vi "SwitchesMirrors Loop.vi"(6 "Used functions":bool, 8 "error in":errorcluster, 9 "IBM OptoElectroMechanics Configuration":T1={"Parameter Analizer"={"Parameter Analyzer VISA Session"="COM1", "Sweeping Time Parameters"={"Integration Time"=0, "Short Integration Time (s)"=1.0, "Long Integration Time (s)"=0.0, "Wait Time Parameter"=1.0}, "Acquisition Mode"=enum."Sweeping Mode", "Status Polling Time (ms)"=0, "Comment"="Test VI", "SMU 1 - Sweeping"={"Start / Offset"=0.0, "Stop / Ratio"=1.0, "Step \n(linear only)"=0.01, "Compliance"=0.1, "Power \nCompliance"=0.0, "Mode"=0, "Function"=0, "Sweep Mode"=FALSE}, "SMU 2 - Sweeping"={"Start / Offset"=0.0, "Stop / Ratio"=1.0, "Step \n(linear only)"=0.01, "Compliance"=0.1, "Power \nCompliance"=0.0, "Mode"=0, "Function"=0, "Sweep Mode"=FALSE}, "SMU 3 - Sweeping"={"Start / Offset"=0.0, "Stop / Ratio"=1.0, "Step \n(linear only)"=0.01, "Compliance"=0.1, "Power \nCompliance"=0.0, "Mode"=0, "Function"=0, "Sweep Mode"=FALSE}, "SMU 4 - Sweeping"={"Start / Offset"=0.0, "Stop / Ratio"=1.0, "Step \n(linear only)"=0.01, "Compliance"=0.1, "Power \nCompliance"=0.0, "Mode"=0, "Function"=0, "Sweep Mode"=FALSE}, "Sweep Spacing"=0, "Range"=0, "SMU1 - Sampling"={"Source"=10.0, "Compliance"=1e-05, "Mode"=0, "Function"=FALSE}, "SMU2 - Sampling"={"Source"=1.0, "Compliance"=1.0, "Mode"=0, "Function"=FALSE}, "SMU3 - Sampling"={"Source"=10.0, "Compliance"=1e-05, "Mode"=0, "Function"=FALSE}, "SMU4 - Sampling"={"Source"=0.1, "Compliance"=60.0, "Mode"=10, "Function"=FALSE}, "Sampling Time Parameters"={"Initial Interval (s)"=0.1, "Number of Samples"=60, "Total Sampling Time (s)"=10.0, "Hold Time (s)"=0.0, "Sampling Mode"=0, "Sampling Time"=0}, "Stop Condition"={"Enable Delay (s)"=0.0, "Name"="", "Threshold"=0.0, "num. of events"=1, "Event"=0, "Stop Condition Enable"=FALSE}}, "Switching Matrix"={"Switching Matrix VISA Session"="GPIB0::18::INSTR", "Connections"=[{"Connections"=[FALSE, FALSE, FALSE, FALSE, FALSE, FALSE, FALSE, FALSE, FALSE, FALSE, FALSE, FALSE], "Connection Type"=enum."Disconnected"}, {"Connections"=[FALSE, FALSE, FALSE, FALSE, FALSE, FALSE, FALSE, FALSE, FALSE, FALSE, FALSE, FALSE], "Connection Type"=enum."Disconnected"}, {"Connections"=[FALSE, FALSE, FALSE, FALSE, FALSE, FALSE, FALSE, FALSE, FALSE, FALSE, FALSE, FALSE], "Connection Type"=enum."Disconnected"}, {"Connections"=[FALSE, FALSE, FALSE, FALSE, FALSE, FALSE, FALSE, FALSE, FALSE, FALSE, FALSE, FALSE], "Connection Type"=enum."Disconnected"}, {"Connections"=[FALSE, FALSE, FALSE, FALSE, FALSE, FALSE, FALSE, FALSE, FALSE, FALSE, FALSE, FALSE], "Connection Type"=enum."Disconnected"}, {"Connections"=[FALSE, FALSE, FALSE, FALSE, FALSE, FALSE, FALSE, FALSE, FALSE, FALSE, FALSE, FALSE], "Connection Type"=enum."Disconnected"}, {"Connections"=[FALSE, FALSE, FALSE, FALSE, FALSE, FALSE, FALSE, FALSE, FALSE, FALSE, FALSE, FALSE], "Connection Type"=enum."Disconnected"}, {"Connections"=[FALSE, FALSE, FALSE, FALSE, FALSE, FALSE, FALSE, FALSE, FALSE, FALSE, FALSE, FALSE], "Connection Type"=enum."Disconnected"}]}, "Stress Control"={"Stress Control VISA Session"="StrainMotor", "Axis"=0, "Motion"=0, "Destination (°)"=0.0, "Speed (°/s)"=4.0, "Position (°)"=25.0}, "Optical Spectrometer"={"Laser Settings"={"Laser Wavelength"=enum."365 nm", "Neutral Density Filter"=enum."100%"}, "Spectrometer Settings"={"Confocal Hole Size (µm)"=0.0, "Grating"=2, "Detector"=enum."InGaAs Array"}, "Acquisition Settings"={"Acquisition Mode"=enum."Multi-Window", "Spectal Position (nm)"=632.0, "From (nm)"=735.0, "To (nm)"=0.0, "Integration Time (s)"=0.0, "Number of Accumulations"=3, "AutoScanning"=FALSE, "Spike Removal"=FALSE}, "Path"=path "C:/07 - Prizes and Awards/Marie Curie Prize/Reply Editors Final NCOMMS(10).docx"}, "Switches & Mirrors"={"Relay VISA Session"="COM1", "Switches"={"Laser"=FALSE, "Video"=FALSE}, "Delays (ms)"={"Laser"=500, "Video"=1500}}, "Camera"={"Settings"={"Pixel clock"=20, "Frame rate"=30.0, "Exposure time"=33.21525, "Master Gain"=0, "Red Gain"=0, "Green Gain"=0, "Blue Gain"=0, "Auto Gain"=FALSE, "White-balance"=FALSE, "Color Correction"=FALSE}}, "XYZ Stage"={"Connection Settings"={"Tango VISA"="", "Baudrate"=57600, "Show Protocol?"=FALSE}, "Manual Control"={"North"=FALSE, "South"=FALSE, "West"=FALSE, "East"=FALSE, "Up"=FALSE, "Down"=FALSE, "Stop"=FALSE, "XY Step"=0.0, "Z step"=0.0}, "Coordinate Control"={"Motion Mode"=enum."Absolute", "Destination [mm]"=[]}}, "AutoFocus"={"Matching Criteria"={"Minimum Score"=700.0, "Color Score Weight"=700.0, "Minimum Contrast"=50, "Match Mode"=0, "Match Feature Mode"=0, "Subpixel Accuracy"=TRUE, "Color Sensitivity"=1, "Search Strategy"=1}, "Z Scan Parameters"={"Z Range"=1380.0, "Resolution"=5000.0, "Initial Direction"=enum."Up", "Focus Threshold"=0.1, "Ascent Constant"=0.1}, "Displacement"=0.0, "Transformation Matrix"=[]}, "Sava Data"={"Workspace Info"={"Device Name"="ProberHead_Tst_C29K3_7(2)", "Device Info"="ProberHead_Tst_C29", "Path"=path "C:/Users/gio/Desktop/ProbeHeadTest"}, "Instrument Configuration"={"Instrument"=enum."Unknown Instrument", "Configuration"="Test Configuration"}, "Stress Motor Position"=0.0, "Electrical Measurement"={"Sequence"=[], "V1"=[], "V2"=[], "V3"=[], "V4"=[], "I1"=[], "I2"=[], "I3"=[], "I4"=[]}, "Optical Spectrum"={"Intensity"=[], "Wavelength"=[], "Energy"=[], "Raman Shift"=[], "Detector Temperature"=0.0}}, "PlotData"={"Sliders"={"Strain Sequence"=0, "Instrument Sequence"=0}, "Measurement"={"Which Instrument?"=enum."No Plot", "Electrical Measurement"={"Sequence"=[], "V1"=[], "V2"=[], "V3"=[], "V4"=[], "I1"=[], "I2"=[], "I3"=[], "I4"=[]}, "Measurement Mode"=enum."Sweeping Mode", "Optical Spectrum"={"Intensity"=[], "Wavelength"=[], "Energy"=[], "Raman Shift"=[], "Detector Temperature"=0.0}}, "Instrument Steps"=[], "Strain Points"=[]}, "Instrument Sequence"={"Caller VI"=enum."User"}, "Strain Measurement"={"Stress Sequence "={"Max Motor Position"=1380.0, "# Intermediate Points"=5000, "Initial Direction"=enum."Tension"}, "Track?"=FALSE}} {"AutoFocus"."Displacement" scale=1.0..1000.0; "AutoFocus"."Z Scan Parameters"."Focus Threshold" min=0.0 max=1000.0 step=1.0 format="%#_2f"; "AutoFocus"."Z Scan Parameters"."Ascent Constant" min=0.0 max=1000.0 step=1.0 format="%#_2f"; "AutoFocus"."Z Scan Parameters"."Resolution" min=0.0 max=1.0 step=0.01 format="%_2g"; "AutoFocus"."Z Scan Parameters"."Z Range" format="%_3g"; "AutoFocus"."Matching Criteria"."Match Mode" items=["Shift Invariant", "Rotation Invariant"]; "AutoFocus"."Matching Criteria"."Match Feature Mode" items=["Color and Shape", "Color", "Shape"]; "AutoFocus"."Matching Criteria"."Color Sensitivity" items=["Low Sensitivity", "Medium Sensitivity", "High Sensitivity"]; "AutoFocus"."Matching Criteria"."Search Strategy" items=["Conservative", "Balance", "Aggressive", "Very Aggressive"]; "XYZ Stage"."Manual Control"."Z step" scale=0.1..10.0; "XYZ Stage"."Manual Control"."XY Step" scale=0.1..1000.0; "Camera"."Settings"."Blue Gain" min=0 max=100 scale=0.0..100.0; "Camera"."Settings"."Green Gain" min=0 max=100 scale=0.0..100.0; "Camera"."Settings"."Red Gain" min=0 max=100 scale=0.0..100.0; "Camera"."Settings"."Master Gain" min=0 max=100 scale=0.0..100.0; "Camera"."Settings"."Exposure time" min=0.101625 max=159.246375 step=0.101625 scale=0.101625..159.246375 scale format="%#.3g"; "Camera"."Settings"."Frame rate" min=2.7455631699174137 max=6.2675785993528725 step=0.000101625 scale=2.7455631699174137..6.2675785993528725 scale format="%^#_3g"; "Camera"."Settings"."Pixel clock" min=5 max=43 scale=5.0..43.0; "PlotData"."Sliders"."Instrument Sequence" scale=0.0..10.0; "PlotData"."Sliders"."Strain Sequence" scale=0.0..10.0; "Strain Measurement"."Stress Sequence"."# Intermediate Points" max=1390; "Parameter Analizer"."Stop Condition"."Event" items=["Value > Threshold", "Value < Threshold", "| Value | > | Threshold |", "| Value | < | Threshold |"]; "Parameter Analizer"."Stop Condition"."Threshold" format="%^.2e"; "Parameter Analizer"."Stop Condition"."Enable Delay (s)" format="%.1f"; "Parameter Analizer"."Sampling Time Parameters"."Sampling Time" items=["Auto (linear only)", "No Limit", "Set Limit"]; "Parameter Analizer"."Sampling Time Parameters"."Sampling Mode" items=["Linear", "Log10", "Log25", "Log50", "Thinned Out"]; "Parameter Analizer"."Sampling Time Parameters"."Hold Time (s)" format="%.4f"; "Parameter Analizer"."Sampling Time Parameters"."Total Sampling Time (s)" format="%.1f"; "Parameter Analizer"."Sampling Time Parameters"."Initial Interval (s)" format="%^.3e"; "Parameter Analizer"."SMU 4 - Sweeping"."Function" items=["Disabled", "Var 1", "Var 2", "Var 1'", "Constant"]; "Parameter Analizer"."SMU 4 - Sweeping"."Mode" items=["V", "I", "V pulse", "I  pulse", "Common"]; "Parameter Analizer"."SMU 4 - Sweeping"."Power \nCompliance" format="%^.2e"; "Parameter Analizer"."SMU 4 - Sweeping"."Compliance" format="%^.2e"; "Parameter Analizer"."SMU 4 - Sweeping"."Step \n(linear only)" format="%^.4e"; "Parameter Analizer"."SMU 4 - Sweeping"."Stop / Ratio" format="%^.4e"; "Parameter Analizer"."SMU 4 - Sweeping"."Start / Offset" format="%^.4e"; "Parameter Analizer"."SMU 3 - Sweeping"."Function" items=["Disabled", "Var 1", "Var 2", "Var 1'", "Constant"]; "Parameter Analizer"."SMU 3 - Sweeping"."Mode" items=["V", "I", "V pulse", "I  pulse", "Common"]; "Parameter Analizer"."SMU 3 - Sweeping"."Power \nCompliance" format="%^.2e"; "Parameter Analizer"."SMU 3 - Sweeping"."Compliance" format="%^.2e"; "Parameter Analizer"."SMU 3 - Sweeping"."Step \n(linear only)" format="%^.4e"; "Parameter Analizer"."SMU 3 - Sweeping"."Stop / Ratio" format="%^.4e"; "Parameter Analizer"."SMU 3 - Sweeping"."Start / Offset" format="%^.4e"; "Parameter Analizer"."SMU 2 - Sweeping"."Function" items=["Disabled", "Var 1", "Var 2", "Var 1'", "Constant"]; "Parameter Analizer"."SMU 2 - Sweeping"."Mode" items=["V", "I", "V pulse", "I  pulse", "Common"]; "Parameter Analizer"."SMU 2 - Sweeping"."Power \nCompliance" format="%^.2e"; "Parameter Analizer"."SMU 2 - Sweeping"."Compliance" format="%^.2e"; "Parameter Analizer"."SMU 2 - Sweeping"."Step \n(linear only)" format="%^.4e"; "Parameter Analizer"."SMU 2 - Sweeping"."Stop / Ratio" format="%^.4e"; "Parameter Analizer"."SMU 2 - Sweeping"."Start / Offset" format="%^.4e"; "Parameter Analizer"."SMU 1 - Sweeping"."Function" items=["Disabled", "Var 1", "Var 2", "Var 1'", "Constant"]; "Parameter Analizer"."SMU 1 - Sweeping"."Mode" items=["V", "I", "V pulse", "I  pulse", "Common"]; "Parameter Analizer"."SMU 1 - Sweeping"."Power \nCompliance" format="%^.2e"; "Parameter Analizer"."SMU 1 - Sweeping"."Compliance" format="%^.2e"; "Parameter Analizer"."SMU 1 - Sweeping"."Step \n(linear only)" format="%^.4e"; "Parameter Analizer"."SMU 1 - Sweeping"."Stop / Ratio" format="%^.4e"; "Parameter Analizer"."SMU 1 - Sweeping"."Start / Offset" format="%^.4e"; "Parameter Analizer"."Sweeping Time Parameters"."Long Integration Time (s)" scale=0.02..2.0; "Parameter Analizer"."Sweeping Time Parameters"."Short Integration Time (s)" scale=8e-05..0.00192; "Parameter Analizer"."Sweeping Time Parameters"."Integration Time" items=["Short", "Long"]; "Parameter Analizer"."Sweeping Time Parameters"."Wait Time Parameter" format="%.1f"; "Parameter Analizer"."SMU4 - Sampling"."Mode" items=["V", "I", "Common"]; "Parameter Analizer"."SMU4 - Sampling"."Compliance" format="%^.2e"; "Parameter Analizer"."SMU4 - Sampling"."Source" format="%^.3e"; "Parameter Analizer"."SMU3 - Sampling"."Mode" items=["V", "I", "Common"]; "Parameter Analizer"."SMU3 - Sampling"."Compliance" format="%^.2e"; "Parameter Analizer"."SMU3 - Sampling"."Source" format="%^.3e"; "Parameter Analizer"."SMU2 - Sampling"."Mode" items=["V", "I", "Common"]; "Parameter Analizer"."SMU2 - Sampling"."Compliance" format="%^.2e"; "Parameter Analizer"."SMU2 - Sampling"."Source" format="%^.3e"; "Parameter Analizer"."SMU1 - Sampling"."Mode" items=["V", "I", "Common"]; "Parameter Analizer"."SMU1 - Sampling"."Compliance" format="%^.2e"; "Parameter Analizer"."SMU1 - Sampling"."Source" format="%^.3e"; "Parameter Analizer"."Range" items=["auto", "fixed", "limited"]; "Parameter Analizer"."Sweep Spacing" items=["linear", "log 10", "log 25", "log 50"]; "Stress Control"."Axis" min=1 max=3; "Stress Control"."Position (°)" format="%.6g"; "Stress Control"."Speed (°/s)" min=0.0 max=4.0 format="%.6f"; "Stress Control"."Destination (°)" min=-2000000000.0 max=2000000000.0 format="%.6f"; "Stress Control"."Motion" items=["Absolute", "Relative"]; "Optical Spectrometer"."Spectrometer Settings"."Grating" items=["1800 l/mm", "150 l/mm"]}, 10 "Message Queues out":T57, 11 "Notifiers":T44) -> (0 "error out":errorcluster)   [LabVIEW 2014]
uses:
  support/Message Queue/All Message Queues.ctl
  support/Message Queue/Message Cluster.ctl
  support/Notifiers/Notifiers.ctl
  support/Message Handler Loop Notifiers.ctl
  Hardware Control/Parameter Analyzer/Parameter Analyzer Notifiers.ctl
  Hardware Control/Switching Matrix/Switching Matrix Notifiers.ctl
  Hardware Control/Stress Control/StressControl Notifiers.ctl
  Hardware Control/Spectrometer/Spectrometer Notifiers.ctl
  Hardware Control/Switches and Mirrors/SwitchesMirrors Notifiers.ctl
  Hardware Control/Camera/Camera Notifiers.ctl
  Hardware Control/XYZ Stage/XYZ Notifications.ctl
  Hardware Control/Autofocus/Autofocus Notifiers.ctl
  Measurements/Optoelectronic Measurement/Optoelectronic Notifiers.ctl
  Measurements/Save Data/SaveData Notifiers.ctl
  Measurements/Instrument Sequence/Instrument Sequence Notifiers.ctl
  support/Configuration/Configuration.ctl
  Hardware Control/Parameter Analyzer/Parameter Analyzer Config.ctl
  Hardware Control/Parameter Analyzer/Parameter Analyzer Integration Parameters.ctl
  Hardware Control/Parameter Analyzer/Parameter Analyzer SMU Sweeping.ctl
  Hardware Control/Parameter Analyzer/Parameter Analyzer Sweep Spacing.ctl
  Hardware Control/Parameter Analyzer/Parameter Analyzer SMU Range.ctl
  Hardware Control/Parameter Analyzer/Parameter Analyzer SMU Sampling.ctl
  Hardware Control/Parameter Analyzer/Parameter Analyzer Sampling Parameters.ctl
  Hardware Control/Parameter Analyzer/Parameter Analyzer Stop Sampling Conditions.ctl
  Hardware Control/Switching Matrix/Switching Matrix Config.ctl
  Hardware Control/Stress Control/StressControl Config.ctl
  Hardware Control/Spectrometer/Spectrometer Config.ctl
  Hardware Control/Spectrometer/Laser Settings.ctl
  Hardware Control/Spectrometer/Laser.ctl
  Hardware Control/Spectrometer/Filter.ctl
  Hardware Control/Spectrometer/Grating Detector Settings.ctl
  Hardware Control/Spectrometer/Grating.ctl
  Hardware Control/Spectrometer/Detector.ctl
  Hardware Control/Spectrometer/Acquisition Settings.ctl
  Hardware Control/Switches and Mirrors/SwitchesMirrors Config.ctl
  Hardware Control/Switches and Mirrors/SwitchesMirrors Status.ctl
  Hardware Control/Camera/Camera Config.ctl
  Hardware Control/Camera/Camera Settings.ctl
  Hardware Control/XYZ Stage/XYZ Config.ctl
  Hardware Control/XYZ Stage/XYZ Connection Settings.ctl
  Hardware Control/XYZ Stage/XYZ Stage Control.ctl
  Hardware Control/XYZ Stage/XYZ Coordinate Control.ctl
  Hardware Control/Autofocus/AutoFocus Config.ctl
  Hardware Control/Autofocus/ZScan.ctl
  <vilib>/Analysis/Matrix/Datatypes/RealMatrix.ctl
  Measurements/Save Data/SaveData Config.ctl
  Measurements/Save Data/SaveData Workspace Info.ctl
  Measurements/Save Data/SaveData Instrument Configuration.ctl
  Measurements/Instrument Sequence/Instrument List.ctl
  Hardware Control/Spectrometer/Spectral Data.ctl
  Measurements/Plot Data/PlotData Config.ctl
  Measurements/Plot Data/Measurement.ctl
  Measurements/Plot Data/WhichInstrument.ctl
  Hardware Control/Parameter Analyzer/Electrical Data.ctl
  Measurements/Instrument Sequence/Instrument Steps.ctl
  Measurements/Instrument Sequence/Action.ctl
  Measurements/Instrument Sequence/Instrument Sequence Config.ctl
  Measurements/Strain Measurement/Strain Measurement Config.ctl
  Hardware Control/Switches and Mirrors/SwitchesMirrors Functions.ctl
  support/Message Queue/Message Queue.lvlib
  <vilib>/Analysis/Matrix/NI_Matrix.lvlib
panel:
  # "LICENSED MATERIALS – PROPERTY OF IBM\nCopyright IBM Corp. 2016,\nALL RIGHTS RESERVED"
  # "XY"
  # "Z"
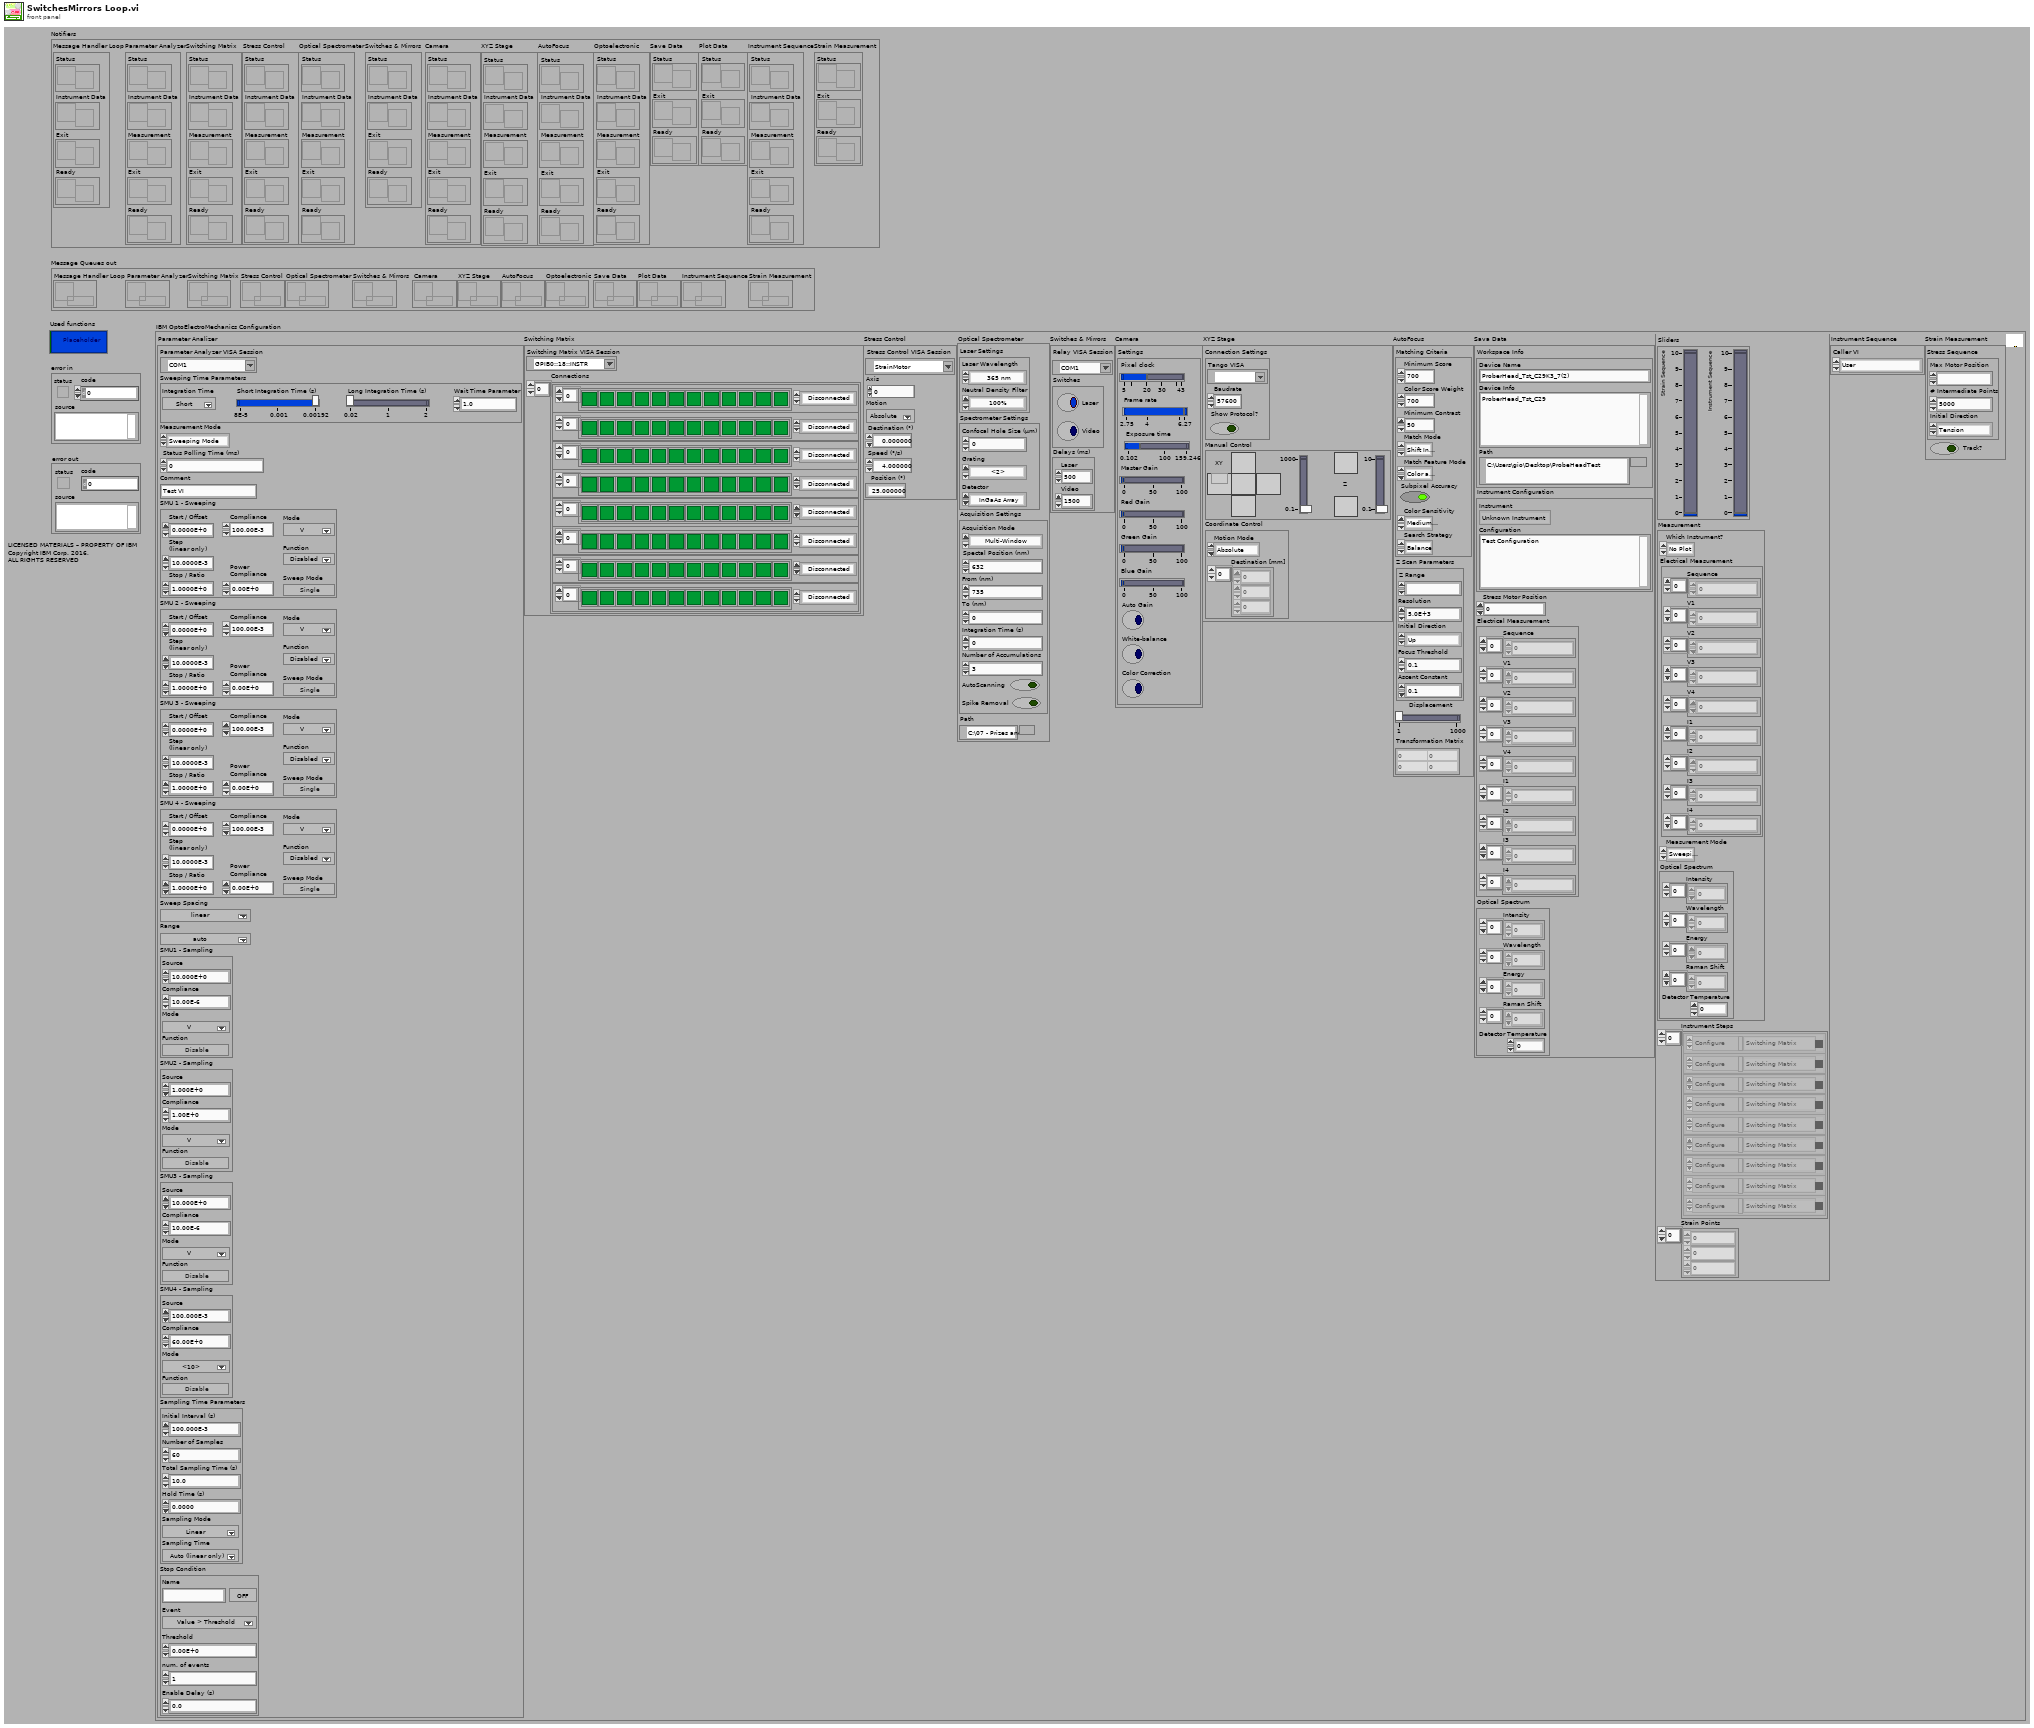
[diagram p1: front panel]
types:
  T1 = typedef "Configuration.ctl" = cluster{"Parameter Analizer":T2, "Switching Matrix":T10, "Stress Control":T11, "Optical Spectrometer":T12, "Switches & Mirrors":T20, "Camera":T22, "XYZ Stage":T24, "AutoFocus":T28, "Sava Data":T31, "PlotData":T36, "Instrument Sequence":T42, "Strain Measurement":T43}
  T2 = typedef "Parameter Analyzer Config.ctl" = cluster{"Parameter Analyzer VISA Session":refnum<visa-resource-name>, "Sweeping Time Parameters":T3, "Acquisition Mode":enum32{"Sweeping Mode", "Sampling Mode"}, "Status Polling Time (ms)":u32, "Comment":string, "SMU 1 - Sweeping":T4, "SMU 2 - Sweeping":T4, "SMU 3 - Sweeping":T4, "SMU 4 - Sweeping":T4, "Sweep Spacing":T5, "Range":T6, "SMU1 - Sampling":T7, "SMU2 - Sampling":T7, "SMU3 - Sampling":T7, "SMU4 - Sampling":T7, "Sampling Time Parameters":T8, "Stop Condition":T9}
  T3 = typedef "Parameter Analyzer Integration Parameters.ctl" = cluster{"Integration Time":u32, "Short Integration Time (s)":dbl, "Long Integration Time (s)":dbl, "Wait Time Parameter":dbl}
  T4 = typedef "Parameter Analyzer SMU Sweeping.ctl" = cluster{"Start / Offset":dbl, "Stop / Ratio":dbl, "Step \n(linear only)":dbl, "Compliance":dbl, "Power \nCompliance":dbl, "Mode":u32, "Function":i32, "Sweep Mode":bool}
  T5 = typedef "Parameter Analyzer Sweep Spacing.ctl" = u16
  T6 = typedef "Parameter Analyzer SMU Range.ctl" = u16
  T7 = typedef "Parameter Analyzer SMU Sampling.ctl" = cluster{"Source":dbl, "Compliance":dbl, "Mode":u32, "Function":bool}
  T8 = typedef "Parameter Analyzer Sampling Parameters.ctl" = cluster{"Initial Interval (s)":dbl, "Number of Samples":i32, "Total Sampling Time (s)":dbl, "Hold Time (s)":dbl, "Sampling Mode":i32, "Sampling Time":i32}
  T9 = typedef "Parameter Analyzer Stop Sampling Conditions.ctl" = cluster{"Enable Delay (s)":dbl, "Name":string, "Threshold":dbl, "num. of events":i32, "Event":i32, "Stop Condition Enable":bool}
  T10 = typedef "Switching Matrix Config.ctl" = cluster{"Switching Matrix VISA Session":refnum<visa-resource-name>, "Connections":cluster{"Connections":bool[], "Connection Type":enum16{"Disconnected", "Make - Break", "Break - Make"}}[]}
  T11 = typedef "StressControl Config.ctl" = cluster{"Stress Control VISA Session":refnum<visa-resource-name>, "Axis":i32, "Motion":u16, "Destination (°)":dbl, "Speed (°/s)":dbl, "Position (°)":dbl}
  T12 = typedef "Spectrometer Config.ctl" = cluster{"Laser Settings":T13, "Spectrometer Settings":T16, "Acquisition Settings":T19, "Path":path}
  T13 = typedef "Laser Settings.ctl" = cluster{"Laser Wavelength":T14, "Neutral Density Filter":T15}
  T14 = typedef "Laser.ctl" = enum16{"633 nm", "784 nm", "532 nm", "365 nm"}
  T15 = typedef "Filter.ctl" = enum16{"100%", "50%", "25%", "10%", "1%", "0.1%", "0.01%"}
  T16 = typedef "Grating Detector Settings.ctl" = cluster{"Confocal Hole Size (µm)":dbl, "Grating":T17, "Detector":T18}
  T17 = typedef "Grating.ctl" = u16
  T18 = typedef "Detector.ctl" = enum16{"InGaAs Array", "Silicon CCD"}
  T19 = typedef "Acquisition Settings.ctl" = cluster{"Acquisition Mode":enum16{"Single Window", "Multi-Window"}, "Spectal Position (nm)":dbl, "From (nm)":dbl, "To (nm)":dbl, "Integration Time (s)":dbl, "Number of Accumulations":i32, "AutoScanning":bool, "Spike Removal":bool}
  T20 = typedef "SwitchesMirrors Config.ctl" = cluster{"Relay VISA Session":refnum<visa-resource-name>, "Switches":T21, "Delays (ms)":cluster{"Laser":u32, "Video":u32}}
  T21 = typedef "SwitchesMirrors Status.ctl" = cluster{"Laser":bool, "Video":bool}
  T22 = typedef "Camera Config.ctl" = cluster{"Settings":T23}
  T23 = typedef "Camera Settings.ctl" = cluster{"Pixel clock":i32, "Frame rate":dbl, "Exposure time":dbl, "Master Gain":i32, "Red Gain":i32, "Green Gain":i32, "Blue Gain":i32, "Auto Gain":bool, "White-balance":bool, "Color Correction":bool}
  T24 = typedef "XYZ Config.ctl" = cluster{"Connection Settings":T25, "Manual Control":T26, "Coordinate Control":T27}
  T25 = typedef "XYZ Connection Settings.ctl" = cluster{"Tango VISA":refnum<visa-resource-name>, "Baudrate":i32, "Show Protocol?":bool}
  T26 = typedef "XYZ Stage Control.ctl" = cluster{"North":bool, "South":bool, "West":bool, "East":bool, "Up":bool, "Down":bool, "Stop":bool, "XY Step":dbl, "Z step":dbl}
  T27 = typedef "XYZ Coordinate Control.ctl" = cluster{"Motion Mode":enum16{"Absolute", "Relative"}, "Destination [mm]":dbl[]}
  T28 = typedef "AutoFocus Config.ctl" = cluster{"Matching Criteria":cluster{"Minimum Score":sgl, "Color Score Weight":sgl, "Minimum Contrast":i32, "Match Mode":u32, "Match Feature Mode":u32, "Subpixel Accuracy":bool, "Color Sensitivity":u32, "Search Strategy":u32}, "Z Scan Parameters":T29, "Displacement":dbl, "Transformation Matrix":T30}
  T29 = typedef "ZScan.ctl" = cluster{"Z Range":ext, "Resolution":dbl, "Initial Direction":enum16{"Up", "Down"}, "Focus Threshold":dbl, "Ascent Constant":dbl}
  T30 = typedef "NI_Matrix.lvlib/RealMatrix.ctl" = dbl[][]
  T31 = typedef "SaveData Config.ctl" = cluster{"Workspace Info":T32, "Instrument Configuration":T33, "Stress Motor Position":dbl, "Electrical Measurement":cluster{"Sequence":dbl[], "V1":dbl[], "V2":dbl[], "V3":dbl[], "V4":dbl[], "I1":dbl[], "I2":dbl[], "I3":dbl[], "I4":dbl[]}, "Optical Spectrum":T35}
  T32 = typedef "SaveData Workspace Info.ctl" = cluster{"Device Name":string, "Device Info":string, "Path":path}
  T33 = typedef "SaveData Instrument Configuration.ctl" = cluster{"Instrument":T34, "Configuration":string}
  T34 = typedef "Instrument List.ctl" = enum32{"Unknown Instrument", "Switching Matrix", "Parameter Analyzer", "Optical Spectrometer", "Optoelectronic", "Autofocus"}
  T35 = typedef "Spectral Data.ctl" = cluster{"Intensity":dbl[], "Wavelength":dbl[], "Energy":dbl[], "Raman Shift":dbl[], "Detector Temperature":dbl}
  T36 = typedef "PlotData Config.ctl" = cluster{"Sliders":cluster{"Strain Sequence":i32, "Instrument Sequence":i32}, "Measurement":T37, "Instrument Steps":T40, "Strain Points":dbl[]}
  T37 = typedef "Measurement.ctl" = cluster{"Which Instrument?":T38, "Electrical Measurement":T39, "Measurement Mode":enum16{"Sweeping Mode", "Sampling Mode"}, "Optical Spectrum":T35}
  T38 = typedef "WhichInstrument.ctl" = enum16{"No Plot", "Spectrometer", "Parameter Analyzer", "Optoelectronic"}
  T39 = typedef "Electrical Data.ctl" = cluster{"Sequence":dbl[], "V1":dbl[], "V2":dbl[], "V3":dbl[], "V4":dbl[], "I1":dbl[], "I2":dbl[], "I3":dbl[], "I4":dbl[]}
  T40 = typedef "Instrument Steps.ctl" = cluster{"Action":T41, "Configuration":variant, "Instrument":T34, "Status":enum8{"False", "True", "Mixed"}}[]
  T41 = typedef "Action.ctl" = enum32{"Configure", "Measure"}
  T42 = typedef "Instrument Sequence Config.ctl" = cluster{"Caller VI":enum16{"User", "Stress Measurement VI"}}
  T43 = typedef "Strain Measurement Config.ctl" = cluster{"Stress Sequence ":cluster{"Max Motor Position":ext, "# Intermediate Points":u32, "Initial Direction":enum16{"Tension", "Compression"}}, "Track?":bool}
  T44 = typedef "Notifiers.ctl" = cluster{"Message Handler Loop":T45, "Parameter Analyzer":T46, "Switching Matrix":T47, "Stress Control":T48, "Optical Spectrometer":T49, "Switches & Mirrors":T50, "Camera":T51, "XYZ Stage":T52, "AutoFocus":T53, "Optoelectronic":T54, "Save Data":T55, "Plot Data":T55, "Instrument Sequence":T56, "Strain Measurement":cluster{"Status":refnum<notifier>, "Exit":refnum<notifier>, "Ready":refnum<notifier>}}
  T45 = typedef "Message Handler Loop Notifiers.ctl" = cluster{"Status":refnum<notifier>, "Instrument Data":refnum<notifier>, "Exit":refnum<notifier>, "Ready":refnum<notifier>}
  T46 = typedef "Parameter Analyzer Notifiers.ctl" = cluster{"Status":refnum<notifier>, "Instrument Data":refnum<notifier>, "Measurement":refnum<notifier>, "Exit":refnum<notifier>, "Ready":refnum<notifier>}
  T47 = typedef "Switching Matrix Notifiers.ctl" = cluster{"Status":refnum<notifier>, "Instrument Data":refnum<notifier>, "Measurement":refnum<notifier>, "Exit":refnum<notifier>, "Ready":refnum<notifier>}
  T48 = typedef "StressControl Notifiers.ctl" = cluster{"Status":refnum<notifier>, "Instrument Data":refnum<notifier>, "Measurement":refnum<notifier>, "Exit":refnum<notifier>, "Ready":refnum<notifier>}
  T49 = typedef "Spectrometer Notifiers.ctl" = cluster{"Status":refnum<notifier>, "Instrument Data":refnum<notifier>, "Measurement":refnum<notifier>, "Exit":refnum<notifier>, "Ready":refnum<notifier>}
  T50 = typedef "SwitchesMirrors Notifiers.ctl" = cluster{"Status":refnum<notifier>, "Instrument Data":refnum<notifier>, "Exit":refnum<notifier>, "Ready":refnum<notifier>}
  T51 = typedef "Camera Notifiers.ctl" = cluster{"Status":refnum<notifier>, "Instrument Data":refnum<notifier>, "Measurement":refnum<notifier>, "Exit":refnum<notifier>, "Ready":refnum<notifier>}
  T52 = typedef "XYZ Notifications.ctl" = cluster{"Status":refnum<notifier>, "Instrument Data":refnum<notifier>, "Measurement":refnum<notifier>, "Exit":refnum<notifier>, "Ready":refnum<notifier>}
  T53 = typedef "Autofocus Notifiers.ctl" = cluster{"Status":refnum<notifier>, "Instrument Data":refnum<notifier>, "Measurement":refnum<notifier>, "Exit":refnum<notifier>, "Ready":refnum<notifier>}
  T54 = typedef "Optoelectronic Notifiers.ctl" = cluster{"Status":refnum<notifier>, "Instrument Data":refnum<notifier>, "Measurement":refnum<notifier>, "Exit":refnum<notifier>, "Ready":refnum<notifier>}
  T55 = typedef "SaveData Notifiers.ctl" = cluster{"Status":refnum<notifier>, "Exit":refnum<notifier>, "Ready":refnum<notifier>}
  T56 = typedef "Instrument Sequence Notifiers.ctl" = cluster{"Status":refnum<notifier>, "Instrument Data":refnum<notifier>, "Measurement":refnum<notifier>, "Exit":refnum<notifier>, "Ready":refnum<notifier>}
  T57 = typedef "Message Queue.lvlib/All Message Queues.ctl" = cluster{"Message Handler Loop":refnum<queue>, "Parameter Analyzer":refnum<queue>, "Switching Matrix":refnum<queue>, "Stress Control":refnum<queue>, "Optical Spectrometer":refnum<queue>, "Switches & Mirrors":refnum<queue>, "Camera":refnum<queue>, "XYZ Stage":refnum<queue>, "AutoFocus":refnum<queue>, "Optoelectronic":refnum<queue>, "Save Data":refnum<queue>, "Plot Data":refnum<queue>, "Instrument Sequence":refnum<queue>, "Strain Measurement":refnum<queue>}
  T58 = typedef "SwitchesMirrors Data.ctl" = cluster{"Configuration":T20, "Refnums":T59, "Initialize":T60}
  T59 = typedef "SwitchesMirrors Refnum.ctl" = cluster{"Instrument Status":refnum<vi>, "Laser":refnum<vi>, "Video":refnum<vi>, "Relay VISA":refnum<vi>}
  T60 = typedef "SwitchesMirrors Initialize.ctl" = cluster{"Update Refnums":bool, "Connect":bool, "Set Configuration":bool}
  T61 = typedef "SwitchesMirrors Functions.ctl" = enum16{"Connect", "Get Configuration", "Set Configuration", "Update Refnums", "Disconnect"}
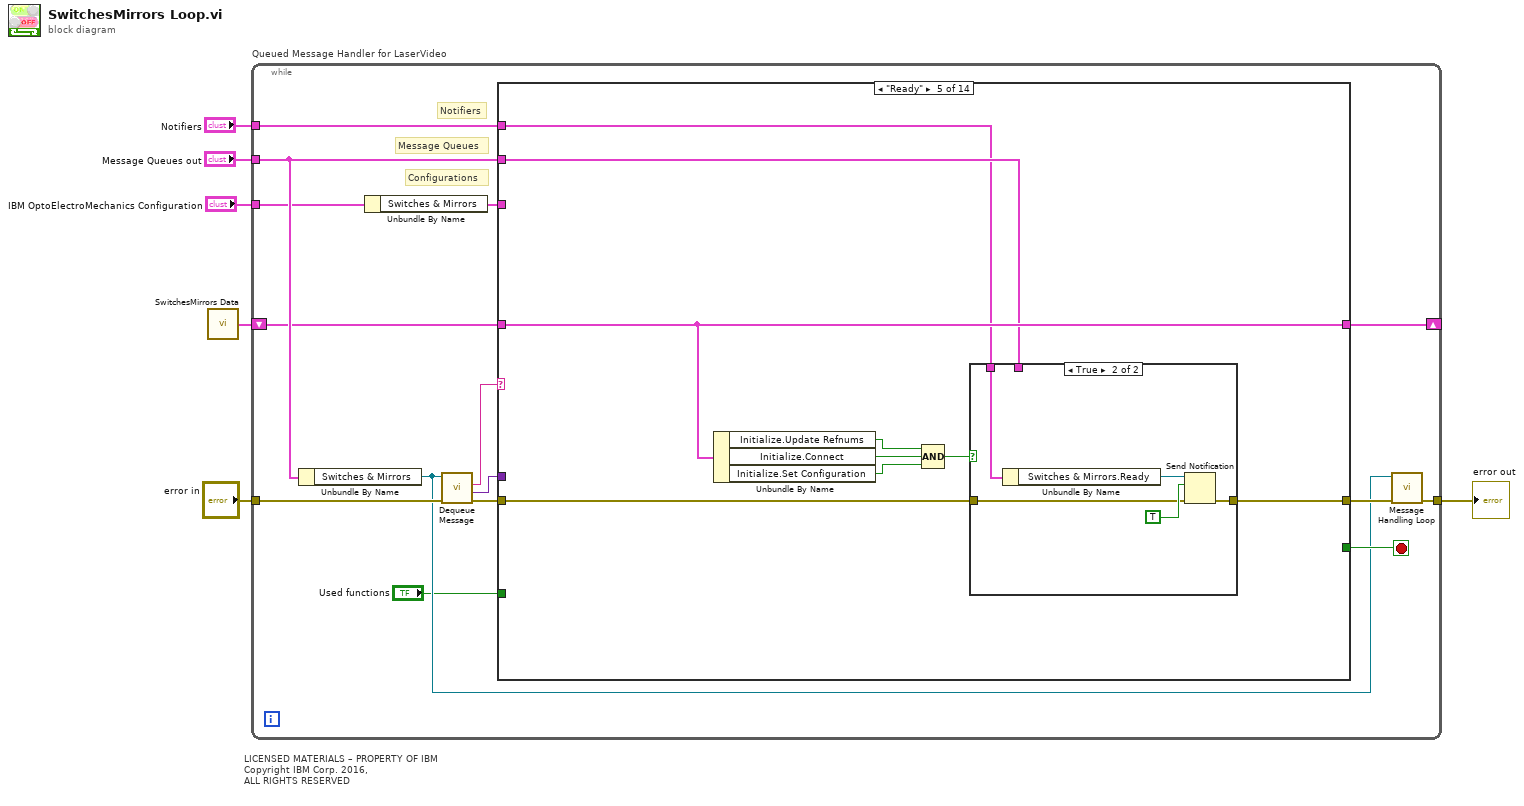
[diagram p0: block diagram]
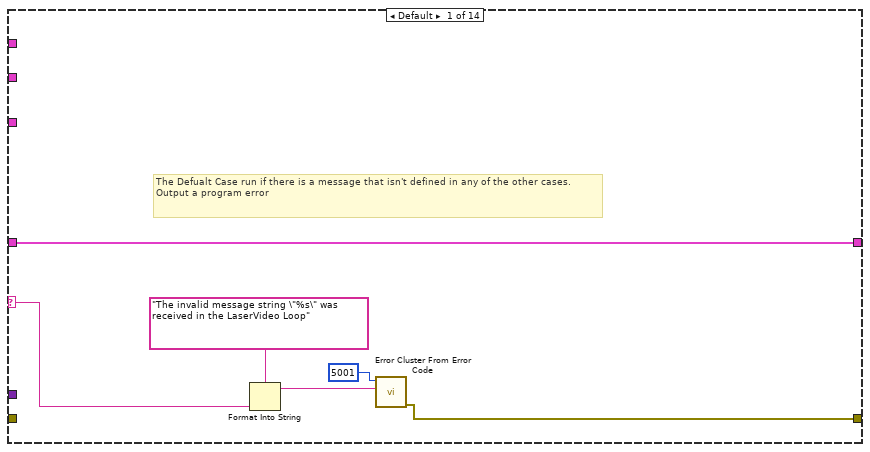
[diagram p2: hidden frame]
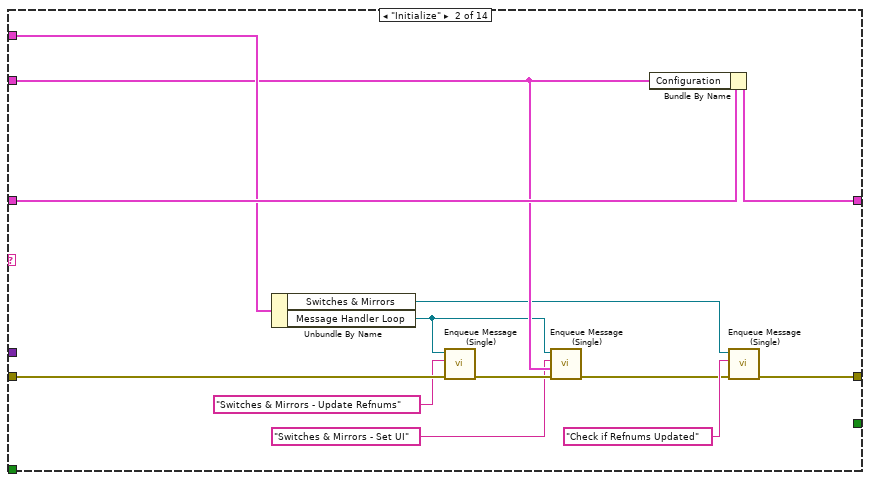
[diagram p3: hidden frame]
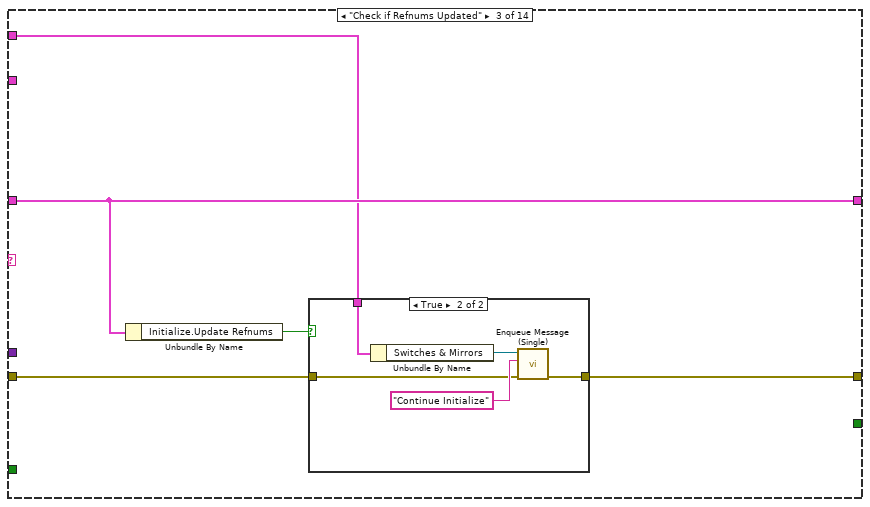
[diagram p4: hidden frame]
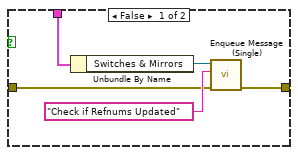
[diagram p5: hidden frame]
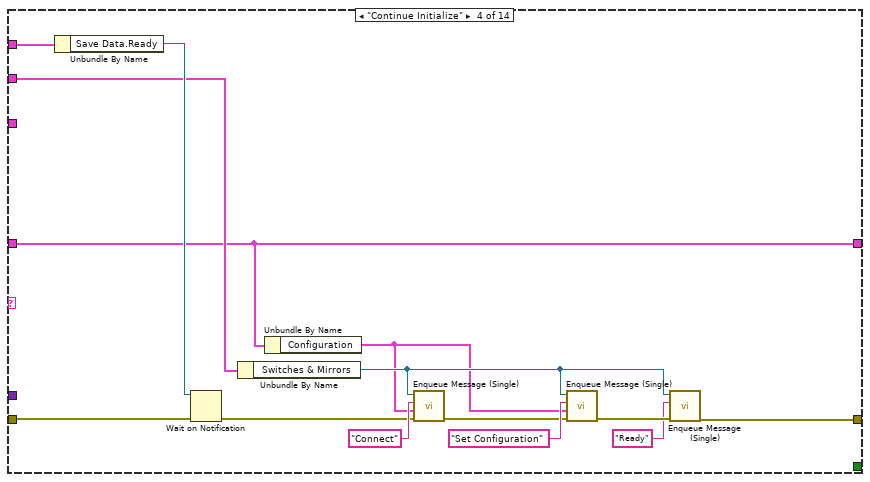
[diagram p6: hidden frame]
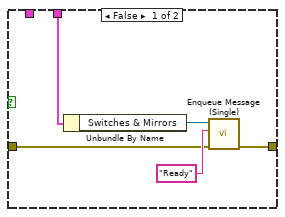
[diagram p7: hidden frame]
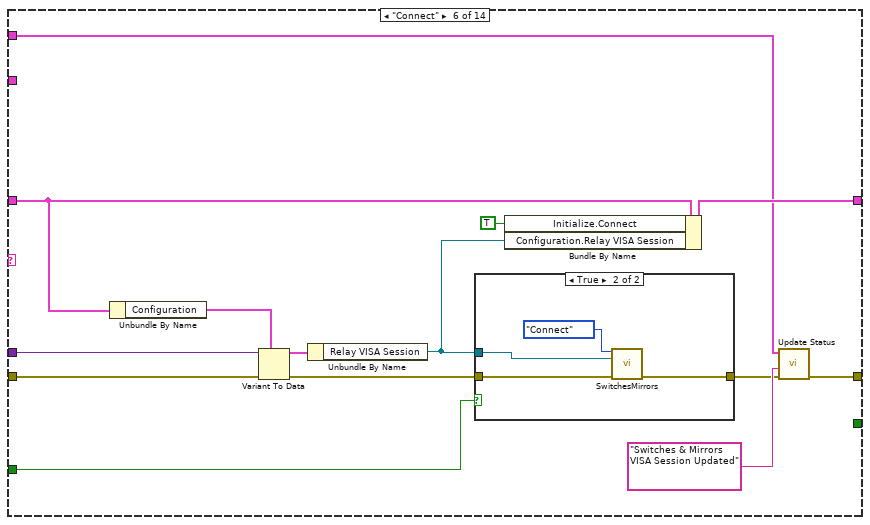
[diagram p8: hidden frame]
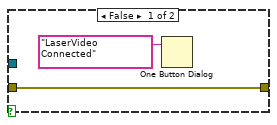
[diagram p9: hidden frame]
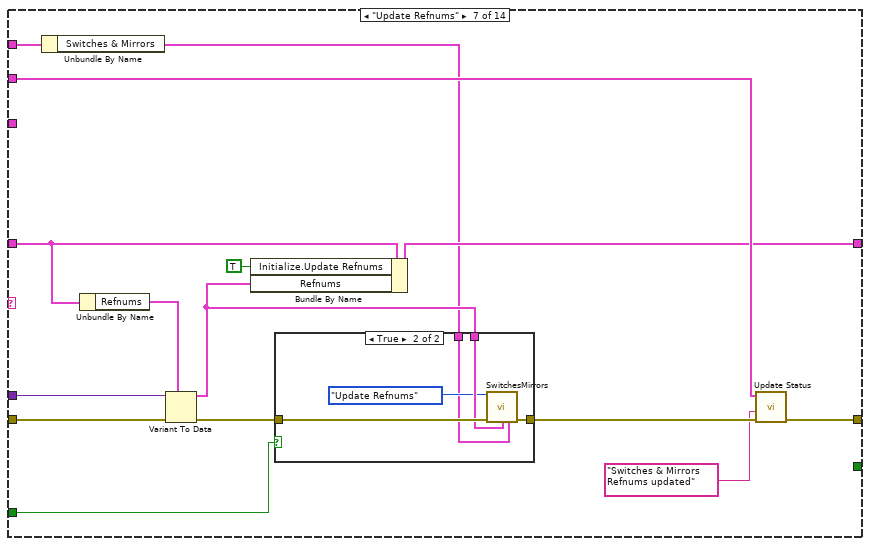
[diagram p10: hidden frame]
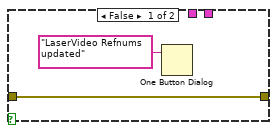
[diagram p11: hidden frame]
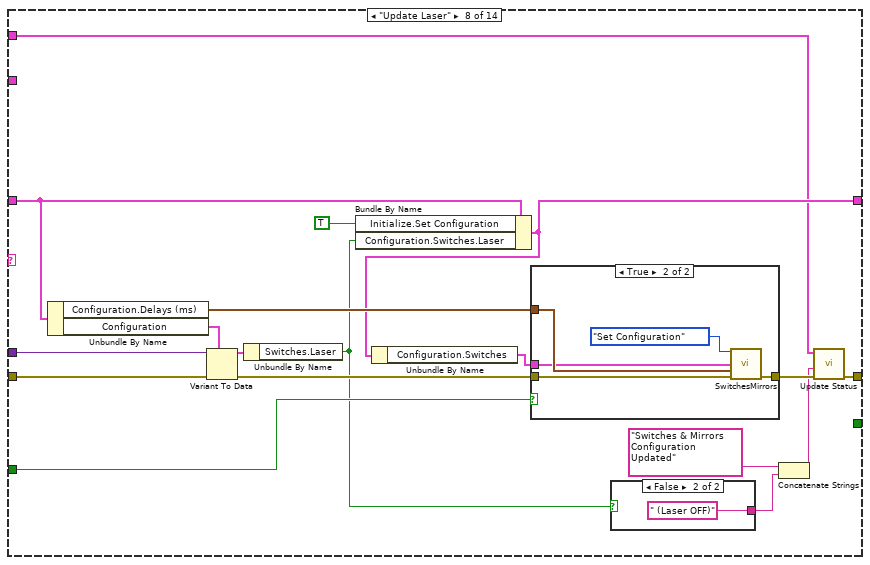
[diagram p12: hidden frame]
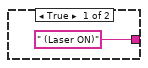
[diagram p13: hidden frame]
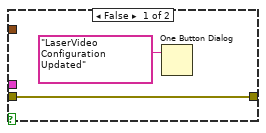
[diagram p14: hidden frame]
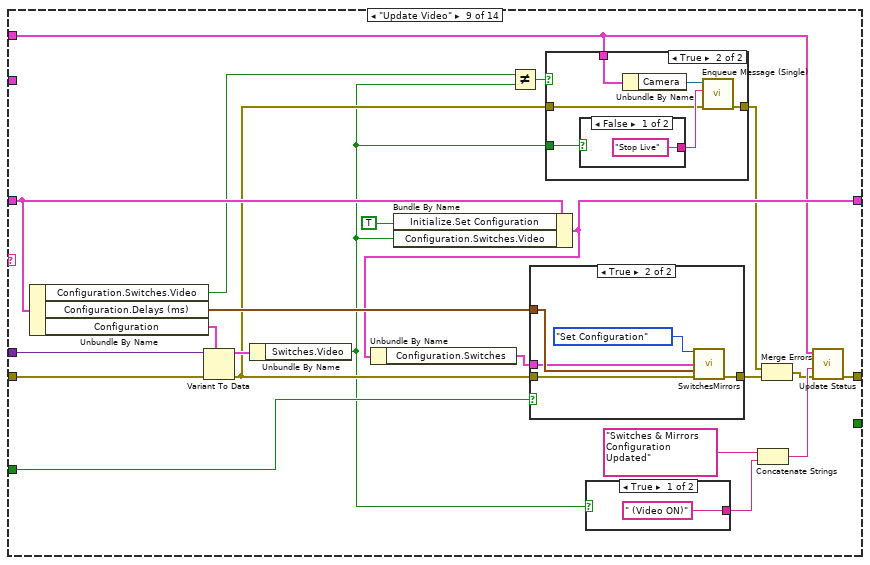
[diagram p15: hidden frame]
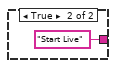
[diagram p17: hidden frame]
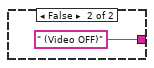
[diagram p18: hidden frame]
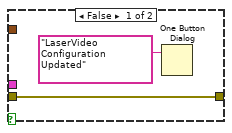
[diagram p19: hidden frame]
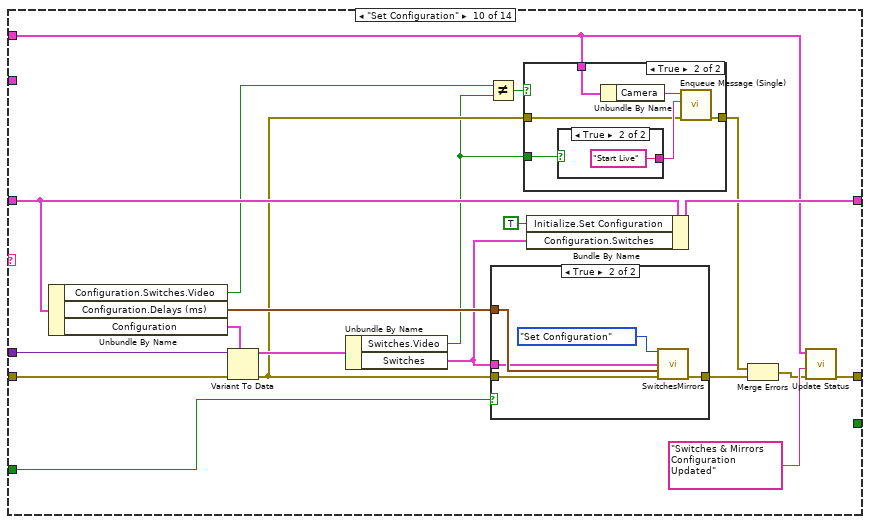
[diagram p20: hidden frame]
diagram:
  # "LICENSED MATERIALS – PROPERTY OF IBM\nCopyright IBM Corp. 2016,\nALL RIGHTS RESERVED"
  n1 = call "SwitchesMirrors Data.vi"() -> ("LaserVideo Data"=w1:T58)
  n2 = while "Queued Message Handler for LaserVideo" {
    tunnel: "error in" -> [w21]
    tunnel: [w13] -> w2
    tunnel: "Message Queues out" -> [w17]
    tunnel: "Notifiers" -> [w16]
    tunnel: "IBM OptoElectroMechanics Configuration" -> [w11]
    shift-right: [w7] -> _
    shift-left: w1 -> [w8]
    stop <- w15 stop-if-true
    # "Configurations"
    # "Notifiers"
    # "Message Queues"
    n3 = Unbundle By Name(w17) -> ("Switches & Mirrors"=w12:refnum<queue>)
    n4 = Unbundle By Name(w11) -> ("Switches & Mirrors"=w10:T20)
    n5 = call "Dequeue Message.vi"("error in (no error)"=w21, "Message Queue"=w12) -> ("error out"=w20:errorcluster, "Message Data"=w18:variant, "Message"=w19:string)  [unwired: 7 out]
    n6 = case shown="\"Ready\"" w19 {
      selector: w19 -> [w24 _ _ _ _ _ _ _ _ _ _ _ _ _]
      tunnel: w20 -> [_ w39 w43 w60 w72 w102 w121 w146 w178 w216 w237 w256 w274 w285]
      tunnel: [w23 w37 w42 w61 w71 w90 w119 w136 w169 w207 w236 w251 w265 w284] -> w14
      tunnel: w18 -> [_ _ _ _ _ w97 w123 w148 w179 w217 _ w249 _ _]
      tunnel: w17 -> [_ w38 w41 w58 w73 w89 w117 w135 w161 w205 _ w257 w276 _]
      tunnel: w16 -> [_ _ _ w59 w70 _ w111 _ _ _ _ _ w264 w286]
      tunnel: [_ _ _ _ _ _ _ _ _ _ _ _ TRUE ("Priority Message? (F)") _] -> w15
      tunnel: w10 -> [_ w35 _ _ _ _ _ _ _ _ _ _ _ _]
      tunnel: w8 -> [w22 w40 w44 w57 w78 w100 w114 w143 w175 w214 w235 w248 w272 w282]
      tunnel: "Used functions" -> [_ _ _ _ _ w101 w120 w145 w177 w215 w238 _ w275 _]
      tunnel: [w22 w36 w44 w57 w78 w96 w113 w139 w171 w210 w234 w248 w272 w282] -> w7
      frame Default {
        # "The Defualt Case run if there is a message that isn't defined in any of the other cases.\nOutput a program error"
        n7 = Format Into String(format string="The invalid message string \"%s\" was  received in the LaserVideo Loop", w24) -> (resulting string=w26:string)  [unwired: 2 in, 1 out]
        n8 = call <vilib>:"Error Cluster From Error Code.vi"("error message (\"\")"=w26, "error code (0)"=5001) -> ("error out"=w23:errorcluster)  [unwired: 2 in, 5 out]
      }
      frame "Initialize" {
        n9 = Unbundle By Name(w38) -> ("Switches & Mirrors"=w33:refnum<queue>, "Message Handler Loop"=w30:refnum<queue>)
        n10 = call "Enqueue Message (Single).vi"("error in (no error)"=w39, "Message"="Switches & Mirrors - Update Refnums", "Message Queue"=w30) -> ("error out"=w31:errorcluster)  [unwired: 1 in, 7 out]
        n11 = call "Enqueue Message (Single).vi"("error in (no error)"=w31, "Message Data"=w35, "Message"="Switches & Mirrors - Set UI", "Message Queue"=w30) -> ("error out"=w28:errorcluster)  [unwired: 7 out]
        n12 = Bundle By Name(cluster=w40, "Configuration"=w35) -> (w36:T58)
        n13 = call "Enqueue Message (Single).vi"("error in (no error)"=w28, "Message"="Check if Refnums Updated", "Message Queue"=w33) -> ("error out"=w37:errorcluster)  [unwired: 1 in, 7 out]
      }
      frame "Check if Refnums Updated" {
        n14 = Unbundle By Name(w44) -> ("Initialize.Update Refnums"=w45:bool)
        n15 = case shown="True" w45 {
          tunnel: w41 -> [w50 w55]
          tunnel: w43 -> [w47 w52]
          tunnel: [w46 w51] -> w42
          frame False {
            n16 = Unbundle By Name(w50) -> ("Switches & Mirrors"=w49:refnum<queue>)
            n17 = call "Enqueue Message (Single).vi"("error in (no error)"=w47, "Message"="Check if Refnums Updated", "Message Queue"=w49) -> ("error out"=w46:errorcluster)  [unwired: 1 in, 7 out]
          }
          frame True {
            n18 = Unbundle By Name(w55) -> ("Switches & Mirrors"=w54:refnum<queue>)
            n19 = call "Enqueue Message (Single).vi"("error in (no error)"=w52, "Message"="Continue Initialize", "Message Queue"=w54) -> ("error out"=w51:errorcluster)  [unwired: 1 in, 7 out]
          }
        }
      }
      frame "Continue Initialize" {
        n20 = Unbundle By Name(w59) -> ("Save Data.Ready"=w62:refnum<notifier>)
        n21 = Wait on Notification(notifier=w62, error in (no error)=w60) -> (error out=w63:errorcluster)  [unwired: 2 in, 3 out]
        n22 = Unbundle By Name(w58) -> ("Switches & Mirrors"=w68:refnum<queue>)
        n23 = Unbundle By Name(w57) -> ("Configuration"=w56:T20)
        n24 = call "Enqueue Message (Single).vi"("error in (no error)"=w63, "Message Data"=w56, "Message"="Connect", "Message Queue"=w68) -> ("error out"=w65:errorcluster)  [unwired: 7 out]
        n25 = call "Enqueue Message (Single).vi"("error in (no error)"=w65, "Message Data"=w56, "Message"="Set Configuration", "Message Queue"=w68) -> ("error out"=w66:errorcluster)  [unwired: 7 out]
        n26 = call "Enqueue Message (Single).vi"("error in (no error)"=w66, "Message"="Ready", "Message Queue"=w68) -> ("error out"=w61:errorcluster)  [unwired: 1 in, 7 out]
      }
      frame "Ready" {
        n27 = Unbundle By Name(w78) -> ("Initialize.Update Refnums"=w77:bool, "Initialize.Connect"=w76:bool, "Initialize.Set Configuration"=w75:bool)
        n28 = Compound Arithmetic op=AND(w77, w76, w75) -> (w74:bool)
        n29 = case shown="True" w74 {
          tunnel: [w82 w87] -> w71
          tunnel: w73 -> [w81 _]
          tunnel: w72 -> [w79 w84]
          tunnel: w70 -> [_ w86]
          frame False {
            n30 = Unbundle By Name(w81) -> ("Switches & Mirrors"=w80:refnum<queue>)
            n31 = call "Enqueue Message (Single).vi"("error in (no error)"=w79, "Message"="Ready", "Message Queue"=w80) -> ("error out"=w82:errorcluster)  [unwired: 1 in, 7 out]
          }
          frame True {
            n32 = Unbundle By Name(w86) -> ("Switches & Mirrors.Ready"=w85:refnum<notifier>)
            n33 = Send Notification(notification=TRUE, notifier=w85, error in (no error)=w84) -> (error out=w87:errorcluster)  [unwired: 1 out]
          }
        }
      }
      frame "Connect" {
        n34 = Unbundle By Name(w100) -> ("Configuration"=w98:T20)
        n35 = Variant To Data(error in=w102, type=w98, Variant=w97) -> (data=w94:T20, error out=w99:errorcluster)
        n36 = Unbundle By Name(w94) -> ("Relay VISA Session"=w93:refnum<visa-resource-name>)
        n37 = case shown="True" w101 {
          tunnel: w99 -> [w104 w108]
          tunnel: [w104 w107] -> w91
          tunnel: w93 -> [_ w105]
          frame False {
            n38 = One Button Dialog(message="LaserVideo Connected" ("button name (\"OK\")")) -> ()  [unwired: 2 out]
          }
          frame True {
            n39 = call "SwitchesMirrors.vi"("Function"=SwitchesMirrors_Functions."Connect", "Relay VISA Session"=w105, "Error In"=w108) -> ("Error Out"=w107:errorcluster)  [unwired: 11 in, 1 out]
          }
        }
        n40 = Bundle By Name(cluster=w100, "Initialize.Connect"=TRUE, "Configuration.Relay VISA Session"=w93) -> (w96:T58)
        n41 = call "Update Status.vi"("error in"=w91, "String"="Switches & Mirrors VISA Session Updated" ("button name (\"OK\")"), "Message Queues out"=w89) -> ("error out"=w90:errorcluster)  [unwired: 8 out]
      }
      frame "Update Refnums" {
        n42 = Unbundle By Name(w111) -> ("Switches & Mirrors"=w110:T50)
        n43 = Unbundle By Name(w114) -> ("Refnums"=w115:T59)
        n44 = Variant To Data(error in=w121, type=w115, Variant=w123) -> (data=w112:T59, error out=w122:errorcluster)
        n45 = Bundle By Name(cluster=w114, "Initialize.Update Refnums"=TRUE, "Refnums"=w112) -> (w113:T58)
        n46 = case shown="True" w120 {
          tunnel: w112 -> [_ w128]
          tunnel: w122 -> [w125 w129]
          tunnel: [w125 w130] -> w118
          tunnel: w110 -> [_ w126]
          frame False {
            n47 = One Button Dialog(message="LaserVideo Refnums updated" ("button name (\"OK\")")) -> ()  [unwired: 2 out]
          }
          frame True {
            n48 = call "SwitchesMirrors.vi"("Function"=SwitchesMirrors_Functions."Update Refnums", "Error In"=w129, "Refnums"=w128, "Notifiers"=w126) -> ("Error Out"=w130:errorcluster)  [unwired: 10 in, 1 out]
          }
        }
        n49 = call "Update Status.vi"("error in"=w118, "String"="Switches & Mirrors Refnums updated" ("button name (\"OK\")"), "Message Queues out"=w117) -> ("error out"=w119:errorcluster)  [unwired: 8 out]
      }
      frame "Update Laser" {
        n50 = Unbundle By Name(w143) -> ("Configuration.Delays (ms)"=w141:cluster{"Laser":u32, "Video":u32}, "Configuration"=w142:T20)
        n51 = Variant To Data(error in=w146, type=w142, Variant=w148) -> (data=w144:T20, error out=w147:errorcluster)
        n52 = Unbundle By Name(w144) -> ("Switches.Laser"=w131:bool)
        n53 = Bundle By Name(cluster=w143, "Initialize.Set Configuration"=TRUE ("Initialize.Set State"), "Configuration.Switches.Laser"=w131) -> (w139:T58)
        n54 = Unbundle By Name(w139) -> ("Configuration.Switches"=w138:T21)
        n55 = case shown="True" w145 {
          tunnel: w147 -> [w152 w156]
          tunnel: [w152 w157] -> w137
          tunnel: w141 -> [_ w154]
          tunnel: w138 -> [_ w153]
          frame False {
            n56 = One Button Dialog(message="LaserVideo Configuration Updated" ("button name (\"OK\")")) -> ()  [unwired: 2 out]
          }
          frame True {
            n57 = call "SwitchesMirrors.vi"("Function"=SwitchesMirrors_Functions."Set Configuration", "Set Switch"=w153, "Delays (ms)"=w154, "Error In"=w156) -> ("Error Out"=w157:errorcluster)  [unwired: 10 in, 1 out]
          }
        }
        n58 = case shown="False" w131 {
          tunnel: [" (Laser ON)" ("button name (\"OK\")") " (Laser OFF)" ("button name (\"OK\")")] -> w132
          frame True {
          }
          frame False {
          }
        }
        n59 = Concatenate Strings("Switches & Mirrors Configuration Updated" ("button name (\"OK\")"), w132) -> (w133:string)
        n60 = call "Update Status.vi"("error in"=w137, "String"=w133, "Message Queues out"=w135) -> ("error out"=w136:errorcluster)  [unwired: 8 out]
      }
      frame "Update Video" {
        n61 = Unbundle By Name(w175) -> ("Configuration.Switches.Video"=w158:bool, "Configuration.Delays (ms)"=w173:cluster{"Laser":u32, "Video":u32}, "Configuration"=w174:T20)
        n62 = Variant To Data(error in=w178, type=w174, Variant=w179) -> (data=w176:T20, error out=w162:errorcluster)
        n63 = Unbundle By Name(w176) -> ("Switches.Video"=w159:bool)
        n64 = Bundle By Name(cluster=w175, "Initialize.Set Configuration"=TRUE ("Initialize.Set State"), "Configuration.Switches.Video"=w159) -> (w171:T58)
        n65 = Unbundle By Name(w171) -> ("Configuration.Switches"=w170:T21)
        n66 = Not Equal?(x=w158, y=w159) -> (x != y?=w160:bool)
        n67 = case shown="True" w177 {
          tunnel: w162 -> [w192 w196]
          tunnel: [w192 w197] -> w168
          tunnel: w173 -> [_ w194]
          tunnel: w170 -> [_ w193]
          frame False {
            n68 = One Button Dialog(message="LaserVideo Configuration Updated" ("button name (\"OK\")")) -> ()  [unwired: 2 out]
          }
          frame True {
            n69 = call "SwitchesMirrors.vi"("Function"=SwitchesMirrors_Functions."Set Configuration", "Set Switch"=w193, "Delays (ms)"=w194, "Error In"=w196) -> ("Error Out"=w197:errorcluster)  [unwired: 10 in, 1 out]
          }
        }
        n70 = case shown="True" w160 {
          tunnel: w161 -> [_ w186]
          tunnel: w162 -> [w180 w183]
          tunnel: [w180 w182] -> w163
          tunnel: w159 -> [_ w181]
          frame False {
          }
          frame True {
            n71 = case shown="False" w181 {
              tunnel: ["Stop Live" ("Message") "Start Live" ("Message")] -> w185
              frame False {
              }
              frame True {
              }
            }
            n72 = Unbundle By Name(w186) -> ("Camera"=w184:refnum<queue>)
            n73 = call "Enqueue Message (Single).vi"("error in (no error)"=w183, "Message"=w185, "Message Queue"=w184) -> ("error out"=w182:errorcluster)  [unwired: 1 in, 7 out]
          }
        }
        n74 = case shown="True" w159 {
          tunnel: [" (Video ON)" ("button name (\"OK\")") " (Video OFF)" ("button name (\"OK\")")] -> w165
          frame True {
          }
          frame False {
          }
        }
        n75 = Concatenate Strings("Switches & Mirrors Configuration Updated" ("button name (\"OK\")"), w165) -> (w166:string)
        n76 = Merge Errors(w163, w168) -> (w164:errorcluster)
        n77 = call "Update Status.vi"("error in"=w164, "String"=w166, "Message Queues out"=w161) -> ("error out"=w169:errorcluster)  [unwired: 8 out]
      }
      frame "Set Configuration" {
        n78 = Unbundle By Name(w214) -> ("Configuration.Switches.Video"=w199:bool, "Configuration.Delays (ms)"=w212:cluster{"Laser":u32, "Video":u32}, "Configuration"=w213:T20)
        n79 = Variant To Data(error in=w216, type=w213, Variant=w217) -> (data=w209:T20, error out=w204:errorcluster)
        n80 = Unbundle By Name(w209) -> ("Switches.Video"=w200:bool, "Switches"=w198:T21)
        n81 = Not Equal?(x=w199, y=w200) -> (x != y?=w201:bool)
        n82 = case shown="True" w215 {
          tunnel: w204 -> [w228 w232]
          tunnel: [w228 w233] -> w208
          tunnel: w212 -> [_ w230]
          tunnel: w198 -> [_ w229]
          frame False {
            n83 = One Button Dialog(message="LaserVideo Configuration Updated" ("button name (\"OK\")")) -> ()  [unwired: 2 out]
          }
          frame True {
            n84 = call "SwitchesMirrors.vi"("Function"=SwitchesMirrors_Functions."Set Configuration", "Set Switch"=w229, "Delays (ms)"=w230, "Error In"=w232) -> ("Error Out"=w233:errorcluster)  [unwired: 10 in, 1 out]
          }
        }
        n85 = case shown="True" w201 {
          tunnel: w205 -> [_ w224]
          tunnel: w204 -> [w218 w221]
          tunnel: [w218 w220] -> w202
          tunnel: w200 -> [_ w219]
          frame False {
          }
          frame True {
            n86 = case shown="True" w219 {
              tunnel: ["Stop Live" ("Message") "Start Live" ("Message")] -> w223
              frame False {
              }
              frame True {
              }
            }
            n87 = Unbundle By Name(w224) -> ("Camera"=w222:refnum<queue>)
            n88 = call "Enqueue Message (Single).vi"("error in (no error)"=w221, "Message"=w223, "Message Queue"=w222) -> ("error out"=w220:errorcluster)  [unwired: 1 in, 7 out]
          }
        }
        n89 = Bundle By Name(cluster=w214, "Initialize.Set Configuration"=TRUE ("Initialize.Set State"), "Configuration.Switches"=w198) -> (w210:T58)
        n90 = Merge Errors(w202, w208) -> (w203:errorcluster)
        n91 = call "Update Status.vi"("error in"=w203, "String"="Switches & Mirrors Configuration Updated" ("button name (\"OK\")"), "Message Queues out"=w205) -> ("error out"=w207:errorcluster)  [unwired: 8 out]
      }
      frame "Get Configuration" {
        n92 = case shown="True" w238 {
          tunnel: w237 -> [w241 w246]
          tunnel: [w241 w247] -> w236
          tunnel: w235 -> [w239 w244]
          tunnel: [w239 w243] -> w234
          frame False {
            n93 = One Button Dialog(message="LaserVideo Configuration Updated" ("button name (\"OK\")")) -> ()  [unwired: 2 out]
          }
          frame True {
            n94 = call "SwitchesMirrors.vi"("Function"=SwitchesMirrors_Functions."Get Configuration", "Error In"=w246) -> ("Get Switch"=w242:T21, "Error Out"=w247:errorcluster)  [unwired: 12 in]
            n95 = Bundle By Name(cluster=w244, "Configuration.Switches"=w242) -> (w243:T58)
          }
        }
      }
      frame "Error" {
        # "Clear Errors to avoid getting stuck \nin repeating this case"
        # "Add here Cases that are handled \nalready by the Message Handler Loop"
        n96 = Variant To Data(error in=w256, type=errorcluster {"status"=FALSE, "code"=0, "source"=""} ("error out"), Variant=w249) -> (data=w255:errorcluster, error out=w254:errorcluster)
        n97 = Merge Errors(w255, w254) -> (w253:errorcluster)
        n98 = Unbundle By Name(w257) -> ("Message Handler Loop"=w259:refnum<queue>)
        n99 = Unbundle By Name(w253) -> ("code"=w250:i32)
        n100 = case shown="Default" w250 {
          tunnel: w259 -> [w263]
          tunnel: w253 -> [w261]
          tunnel: [w260] -> w252
          frame Default {
            n101 = call "Enqueue Message (Single).vi"("Message Data"=w261, "Message"="Error", "Message Queue"=w263) -> ("error out"=w260:errorcluster)  [unwired: 1 in, 7 out]
          }
        }
        n102 = call <vilib>:"Clear Errors.vi"("error in (no error)"=w252) -> ("error out"=w251:errorcluster)  [unwired: 1 in, 5 out]
      }
      frame "Exit" {
        w268 = TRUE ("Priority Message? (F)")
        # "Stip the VI"
        n103 = case shown="True" w275 {
          tunnel: w274 -> [w278 w280]
          tunnel: [w278 w281] -> w273
          frame False {
          }
          frame True {
            n104 = call "SwitchesMirrors.vi"("Function"=SwitchesMirrors_Functions."Disconnect", "Error In"=w280) -> ("Error Out"=w281:errorcluster)  [unwired: 12 in, 1 out]
          }
        }
        n105 = Unbundle By Name(w276) -> ("Switches & Mirrors"=w277:refnum<queue>)
        n106 = Unbundle By Name(w264) -> ("Switches & Mirrors.Exit"=w267:refnum<notifier>, "Switches & Mirrors.Ready"=w270:refnum<notifier>)
        n107 = Release Queue(queue=w277, error in (no error)=w273) -> (error out=w266:errorcluster)  [unwired: 3 out]
        n108 = Send Notification(notification=w268, notifier=w270, error in (no error)=w266) -> (error out=w269:errorcluster)  [unwired: 1 out]
        n109 = Send Notification(notification=w268, notifier=w267, error in (no error)=w269) -> (error out=w265:errorcluster)  [unwired: 1 out]
      }
      frame "Notify Status" {
        n110 = Unbundle By Name(w286) -> ("Switches & Mirrors.Instrument Data"=w283:refnum<notifier>)
        n111 = Send Notification(notification=w282, notifier=w283, error in (no error)=w285) -> (error out=w284:errorcluster)  [unwired: 1 out]
      }
    }
    n112 = call "Message Handling Loop.vi"("error in (no error)"=w14, "Message Queue"=w12) -> ("dup error in"=w13:errorcluster)  [unwired: 9 out]
  }
  "error out" <- w2
